vi "Load Edit Data Type.vi"(8 "error in":errorcluster, 10 "Data Type":string[](array[string]), 11 "Panel Bounds":T1) -> (0 "error out":errorcluster)   [LabVIEW 2020, in "Data Type Scripting.lvlib"]
doc: "_____\nCreated using DQMH Event Scripter 6.0.0.122."
uses:
  Data Type Scripting.lvlib
  <vilib>/Utility/miscctls.llb/LVRectTypeDef.ctl
  Edit Data Type Argument--cluster.ctl
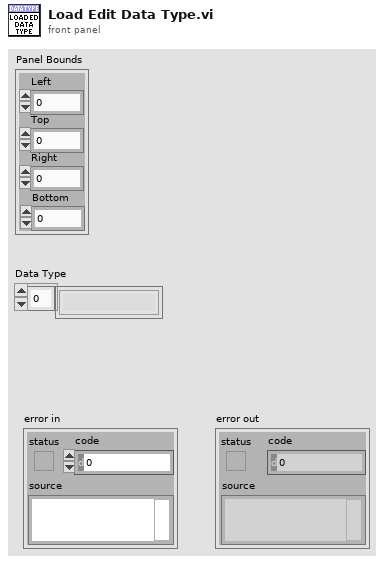
[diagram p1: front panel]
types:
  T1 = typedef "LVRectTypeDef.ctl" = cluster{"Left":i16, "Top":i16, "Right":i16, "Bottom":i16}
  T2 = typedef "Data Type Scripting.lvlib/Edit Data Type Argument--cluster.ctl" = cluster{"Data Type":string[], "Panel Bounds":T1}
  T3 = typedef "Data Type Scripting.lvlib/Request Events--cluster.ctl" = cluster{"Stop Module":refnum<user-event>, "Show Panel":refnum<user-event>, "Hide Panel":refnum<user-event>, "Get Module Execution Status":refnum<user-event>, "Show Diagram":refnum<user-event>, "Load Poly VI":refnum<user-event>, "Get Poly List":refnum<user-event>, "Get Poly Details":refnum<user-event>, "Open Poly VI Window":refnum<user-event>, "Create New Data Type":refnum<user-event>, "Verify New Data Type":refnum<user-event>, "Get List of Data Types":refnum<user-event>, "Remove Data Type":refnum<user-event>, "Open Process Data TypeDef":refnum<user-event>, "Load Edit Data Type":refnum<user-event>, "Close Process Data Type Def":refnum<user-event>}
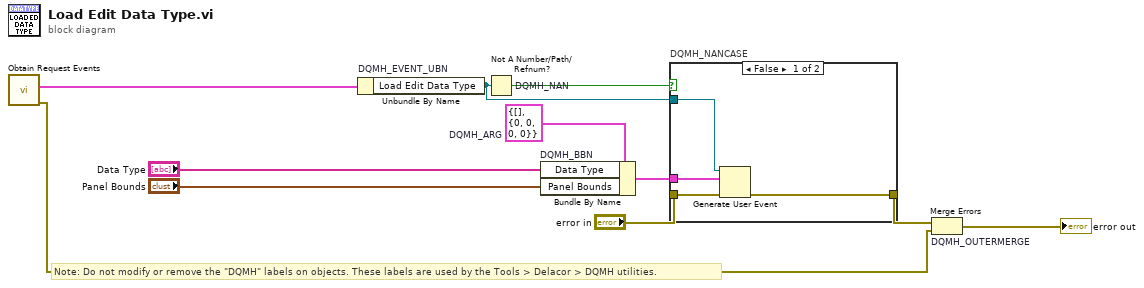
[diagram p0: block diagram]
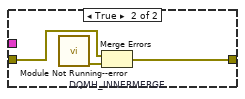
[diagram p2: hidden frame]
diagram:
  w5 = T2 {"Data Type"=[], "Panel Bounds"={"Left"=0, "Top"=0, "Right"=0, "Bottom"=0}}  # DQMH_ARG
  # "Note: Do not modify or remove the \"DQMH\" labels on objects. These labels are used by the Tools > Delacor > DQMH utilities."
  n1 = call "Obtain Request Events.vi"() -> ("error out"=w3:errorcluster, "Data Type Scripting Request Events"=w2:T3)  [unwired: 10 in]
  n2 = Unbundle By Name "DQMH_EVENT_UBN"(w2) -> ("Load Edit Data Type"=w7:refnum<user-event>)
  n3 = Not A Number/Path/Refnum? "DQMH_NAN"(number/path/refnum=w7) -> (NaN/Path/Refnum?=w8:bool)
  n4 = Bundle By Name "DQMH_BBN"(cluster=w5, "Data Type"="Data Type", "Panel Bounds"="Panel Bounds") -> (w9:T2)
  n5 = case "DQMH_NANCASE" shown="False" w8 {
    tunnel: "error in" -> [w15 w18]
    tunnel: [w14 w17] -> w6
    tunnel: w7 -> [w13 _]
    tunnel: w9 -> [w12 _]
    frame False {
      n6 = Generate User Event(user event=w13, event data cluster=w12, error in=w15) -> (error out=w14:errorcluster)  [unwired: 1 in, 1 out]
    }
    frame True {
      n7 = call "Module Not Running--error.vi"() -> ("error out"=w16:errorcluster)  [unwired: 11 in]
      n8 = Merge Errors "DQMH_INNERMERGE"(w18, w16) -> (w17:errorcluster)
    }
  }
  n9 = Merge Errors "DQMH_OUTERMERGE"(w6, w3) -> (→"error out":errorcluster)
